vi "append_array.vi"(1 "array 2":string[][](array[string]), 2 "array 1":string[][](array[string])) -> (0 "appended array":string[][](array[string]))   [LabVIEW 2010]
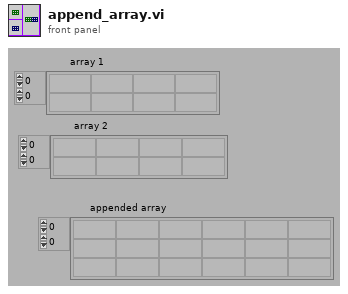
[diagram p1: front panel]
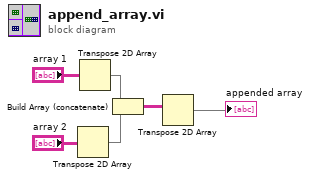
[diagram p0: block diagram]
diagram:
  n1 = Transpose 2D Array(2D array="array 2") -> (transposed array=w4:string[][])
  n2 = Transpose 2D Array(2D array="array 1") -> (transposed array=w5:string[][])
  n3 = Build Array (concatenate)(w5, w4) -> (w2:string[][])
  n4 = Transpose 2D Array(2D array=w2) -> (transposed array=→"appended array":string[][])
